vi "Config_LoadCreate.vi"(7 "Config In":path, 8 "error In":errorcluster, 10 "Configuration Cluster":T1={"General"={"Config.ini"=path "", "Default Logging Path"=path ""}, "Hardware"={"LCR VISA COM"="", "Measure Rate (1/s)"=0, "Reset on Load?"=FALSE, "Measure Profile"=path ""}, "HM8118 Current Profile"={"Bias Profile"={" Bias Source (OFF)"=0, " Bias Type (Voltage)"=0, "Bias Level (0)"=0.0}, "Measurement Profile"={"Operation Mode (0: Auto)"=0, "Circuit Type (2: Auto)"=2, "Manual Range (1:Range 1 and 25 Ohms)"=1, "Auto Range (T: Enable)"=TRUE}, "Signal Profile"={"Frequency (1kHz)"=1000.0, "Measuring Voltage (1V)"=1.0}, "Integration Profile"={"Averaging (0: Off)"=0, "Averaging Number (2)"=2, "Time (100ms)"=100, "Rate (0: Fast)"=0}, "Trigger Profile"={"Trigger Mode (0: Continuous)"=0}}, "HM8118 New Profile"={"Bias Profile"={" Bias Source (OFF)"=0, " Bias Type (Voltage)"=0, "Bias Level (0)"=0.0}, "Measurement Profile"={"Operation Mode (0: Auto)"=0, "Circuit Type (2: Auto)"=2, "Manual Range (1:Range 1 and 25 Ohms)"=1, "Auto Range (T: Enable)"=TRUE}, "Signal Profile"={"Frequency (1kHz)"=1000.0, "Measuring Voltage (1V)"=1.0}, "Integration Profile"={"Averaging (0: Off)"=0, "Averaging Number (2)"=2, "Time (100ms)"=100, "Rate (0: Fast)"=0}, "Trigger Profile"={"Trigger Mode (0: Continuous)"=0}}, "Operation"={"Operation Mode"=enum."Logging", "Status"=""}} {"HM8118 New Profile"."Trigger Profile"."Trigger Mode (0: Continuous)" items=["Continuous", "Manual", "External"]; "HM8118 New Profile"."Integration Profile"."Rate (0: Fast)" items=["Fast", "Medium", "Slow"]; "HM8118 New Profile"."Integration Profile"."Time (100ms)" min=1 max=999; "HM8118 New Profile"."Integration Profile"."Averaging Number (2)" min=2 max=99; "HM8118 New Profile"."Integration Profile"."Averaging (0: Off)" items=["Off", "Normal", "Averaging"]; "HM8118 New Profile"."Signal Profile"."Measuring Voltage (1V)" min=0.05 max=1.5 step=0.01; "HM8118 New Profile"."Signal Profile"."Frequency (1kHz)" min=20.0 max=200000.0; "HM8118 New Profile"."Measurement Profile"."Manual Range (1:Range 1 and 25 Ohms)" items=["Range 1 and 25 Ohms"=1, "Range 2 and 25 Ohms"=2, "Range 3 and 400 Ohms"=3, "Range 4 and 6.4 kOhms"=4, "Range 5 and 100kOhms"=5, "Range 6 and 100kOhms"=6]; "HM8118 New Profile"."Measurement Profile"."Circuit Type (2: Auto)" items=["Series", "Parallel", "Auto"]; "HM8118 New Profile"."Measurement Profile"."Operation Mode (0: Auto)" items=["Auto", "L+Q", "L+R", "C+D", "C+R", "R+Q", "Z+Theta", "Y+Theta", "R+X", "G+B", "N+Theta", "M"]; "HM8118 New Profile"."Bias Profile"."Bias Type (Voltage)" items=["Voltage", "Current"]; "HM8118 New Profile"."Bias Profile"."Bias Source (OFF)" items=["Off", "Internal", "External"]; "HM8118 Current Profile"."Trigger Profile"."Trigger Mode (0: Continuous)" items=["Continuous", "Manual", "External"]; "HM8118 Current Profile"."Integration Profile"."Rate (0: Fast)" items=["Fast", "Medium", "Slow"]; "HM8118 Current Profile"."Integration Profile"."Time (100ms)" min=1 max=999; "HM8118 Current Profile"."Integration Profile"."Averaging Number (2)" min=2 max=99; "HM8118 Current Profile"."Integration Profile"."Averaging (0: Off)" items=["Off", "Normal", "Averaging"]; "HM8118 Current Profile"."Signal Profile"."Measuring Voltage (1V)" min=0.05 max=1.5 step=0.01; "HM8118 Current Profile"."Signal Profile"."Frequency (1kHz)" min=20.0 max=200000.0; "HM8118 Current Profile"."Measurement Profile"."Manual Range (1:Range 1 and 25 Ohms)" items=["Range 1 and 25 Ohms"=1, "Range 2 and 25 Ohms"=2, "Range 3 and 400 Ohms"=3, "Range 4 and 6.4 kOhms"=4, "Range 5 and 100kOhms"=5, "Range 6 and 100kOhms"=6]; "HM8118 Current Profile"."Measurement Profile"."Circuit Type (2: Auto)" items=["Series", "Parallel", "Auto"]; "HM8118 Current Profile"."Measurement Profile"."Operation Mode (0: Auto)" items=["Auto", "L+Q", "L+R", "C+D", "C+R", "R+Q", "Z+Theta", "Y+Theta", "R+X", "G+B", "N+Theta", "M"]; "HM8118 Current Profile"."Bias Profile"."Bias Type (Voltage)" items=["Voltage", "Current"]; "HM8118 Current Profile"."Bias Profile"."Bias Source (OFF)" items=["Off", "Internal", "External"]}, 11 "LCR VISA COM":refnum<visa-resource-name>) -> (0 "error out":errorcluster, 2 "Configuration Cluster Out":T1={"General"={"Config.ini"=path "", "Default Logging Path"=path ""}, "Hardware"={"LCR VISA COM"="", "Measure Rate (1/s)"=0, "Reset on Load?"=FALSE, "Measure Profile"=path ""}, "HM8118 Current Profile"={"Bias Profile"={" Bias Source (OFF)"=0, " Bias Type (Voltage)"=0, "Bias Level (0)"=0.0}, "Measurement Profile"={"Operation Mode (0: Auto)"=0, "Circuit Type (2: Auto)"=2, "Manual Range (1:Range 1 and 25 Ohms)"=1, "Auto Range (T: Enable)"=TRUE}, "Signal Profile"={"Frequency (1kHz)"=1000.0, "Measuring Voltage (1V)"=1.0}, "Integration Profile"={"Averaging (0: Off)"=0, "Averaging Number (2)"=2, "Time (100ms)"=100, "Rate (0: Fast)"=0}, "Trigger Profile"={"Trigger Mode (0: Continuous)"=0}}, "HM8118 New Profile"={"Bias Profile"={" Bias Source (OFF)"=0, " Bias Type (Voltage)"=0, "Bias Level (0)"=0.0}, "Measurement Profile"={"Operation Mode (0: Auto)"=0, "Circuit Type (2: Auto)"=2, "Manual Range (1:Range 1 and 25 Ohms)"=1, "Auto Range (T: Enable)"=TRUE}, "Signal Profile"={"Frequency (1kHz)"=1000.0, "Measuring Voltage (1V)"=1.0}, "Integration Profile"={"Averaging (0: Off)"=0, "Averaging Number (2)"=2, "Time (100ms)"=100, "Rate (0: Fast)"=0}, "Trigger Profile"={"Trigger Mode (0: Continuous)"=0}}, "Operation"={"Operation Mode"=enum."Logging", "Status"=""}} {"HM8118 New Profile"."Trigger Profile"."Trigger Mode (0: Continuous)" items=["Continuous", "Manual", "External"]; "HM8118 New Profile"."Integration Profile"."Rate (0: Fast)" items=["Fast", "Medium", "Slow"]; "HM8118 New Profile"."Integration Profile"."Time (100ms)" min=1 max=999; "HM8118 New Profile"."Integration Profile"."Averaging Number (2)" min=2 max=99; "HM8118 New Profile"."Integration Profile"."Averaging (0: Off)" items=["Off", "Normal", "Averaging"]; "HM8118 New Profile"."Signal Profile"."Measuring Voltage (1V)" min=0.05 max=1.5 step=0.01; "HM8118 New Profile"."Signal Profile"."Frequency (1kHz)" min=20.0 max=200000.0; "HM8118 New Profile"."Measurement Profile"."Manual Range (1:Range 1 and 25 Ohms)" items=["Range 1 and 25 Ohms"=1, "Range 2 and 25 Ohms"=2, "Range 3 and 400 Ohms"=3, "Range 4 and 6.4 kOhms"=4, "Range 5 and 100kOhms"=5, "Range 6 and 100kOhms"=6]; "HM8118 New Profile"."Measurement Profile"."Circuit Type (2: Auto)" items=["Series", "Parallel", "Auto"]; "HM8118 New Profile"."Measurement Profile"."Operation Mode (0: Auto)" items=["Auto", "L+Q", "L+R", "C+D", "C+R", "R+Q", "Z+Theta", "Y+Theta", "R+X", "G+B", "N+Theta", "M"]; "HM8118 New Profile"."Bias Profile"."Bias Type (Voltage)" items=["Voltage", "Current"]; "HM8118 New Profile"."Bias Profile"."Bias Source (OFF)" items=["Off", "Internal", "External"]; "HM8118 Current Profile"."Trigger Profile"."Trigger Mode (0: Continuous)" items=["Continuous", "Manual", "External"]; "HM8118 Current Profile"."Integration Profile"."Rate (0: Fast)" items=["Fast", "Medium", "Slow"]; "HM8118 Current Profile"."Integration Profile"."Time (100ms)" min=1 max=999; "HM8118 Current Profile"."Integration Profile"."Averaging Number (2)" min=2 max=99; "HM8118 Current Profile"."Integration Profile"."Averaging (0: Off)" items=["Off", "Normal", "Averaging"]; "HM8118 Current Profile"."Signal Profile"."Measuring Voltage (1V)" min=0.05 max=1.5 step=0.01; "HM8118 Current Profile"."Signal Profile"."Frequency (1kHz)" min=20.0 max=200000.0; "HM8118 Current Profile"."Measurement Profile"."Manual Range (1:Range 1 and 25 Ohms)" items=["Range 1 and 25 Ohms"=1, "Range 2 and 25 Ohms"=2, "Range 3 and 400 Ohms"=3, "Range 4 and 6.4 kOhms"=4, "Range 5 and 100kOhms"=5, "Range 6 and 100kOhms"=6]; "HM8118 Current Profile"."Measurement Profile"."Circuit Type (2: Auto)" items=["Series", "Parallel", "Auto"]; "HM8118 Current Profile"."Measurement Profile"."Operation Mode (0: Auto)" items=["Auto", "L+Q", "L+R", "C+D", "C+R", "R+Q", "Z+Theta", "Y+Theta", "R+X", "G+B", "N+Theta", "M"]; "HM8118 Current Profile"."Bias Profile"."Bias Type (Voltage)" items=["Voltage", "Current"]; "HM8118 Current Profile"."Bias Profile"."Bias Source (OFF)" items=["Off", "Internal", "External"]}, 3 "LCR VISA COM Out":refnum<visa-resource-name>)   [LabVIEW 2021]
uses:
  Config_Cluster.ctl
  Mode_Enum.ctl
  <vilib>/Utility/config.llb/Read Key (Path).vi
  <vilib>/Utility/config.llb/NI_LVConfig.lvlib
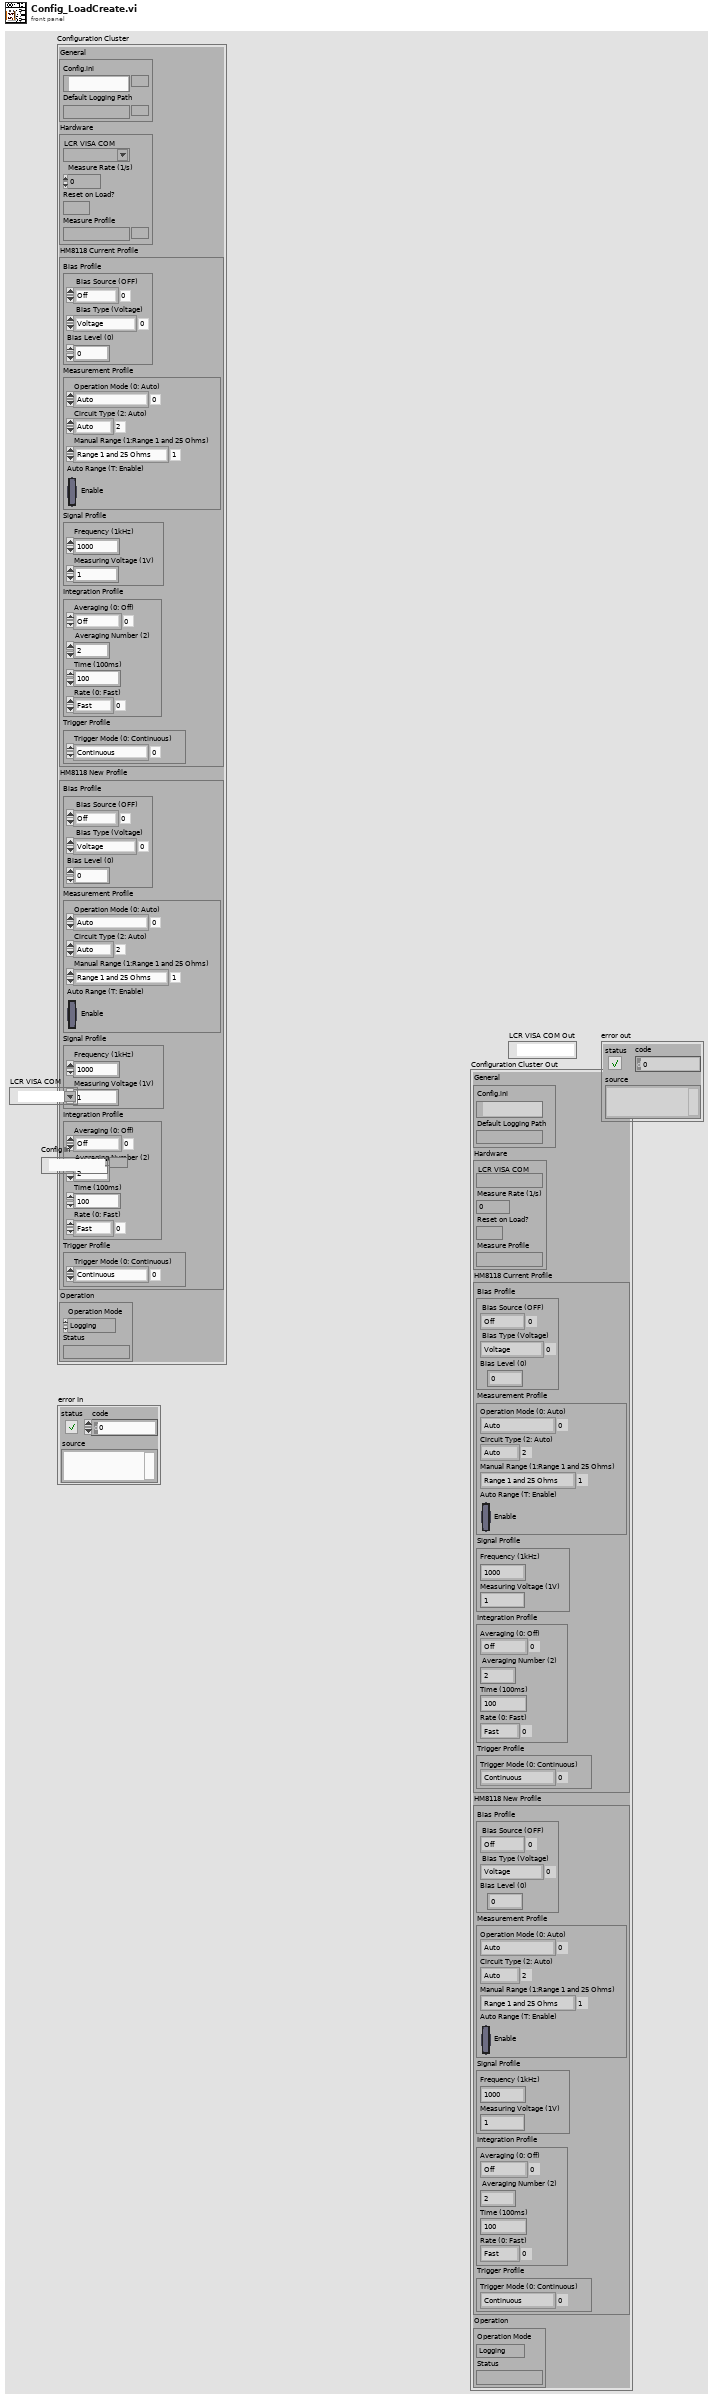
[diagram p1: front panel]
types:
  T1 = typedef "Config_Cluster.ctl" = cluster{"General":cluster{"Config.ini":path, "Default Logging Path":path}, "Hardware":cluster{"LCR VISA COM":refnum<visa-resource-name>, "Measure Rate (1/s)":i32, "Reset on Load?":bool, "Measure Profile":path}, "HM8118 Current Profile":cluster{"Bias Profile":cluster{" Bias Source (OFF)":u8, " Bias Type (Voltage)":u8, "Bias Level (0)":dbl}, "Measurement Profile":cluster{"Operation Mode (0: Auto)":u16, "Circuit Type (2: Auto)":u16, "Manual Range (1:Range 1 and 25 Ohms)":u8, "Auto Range (T: Enable)":bool}, "Signal Profile":cluster{"Frequency (1kHz)":dbl, "Measuring Voltage (1V)":dbl}, "Integration Profile":cluster{"Averaging (0: Off)":u16, "Averaging Number (2)":i32, "Time (100ms)":i32, "Rate (0: Fast)":u16}, "Trigger Profile":cluster{"Trigger Mode (0: Continuous)":u16}}, "HM8118 New Profile":cluster{"Bias Profile":cluster{" Bias Source (OFF)":u8, " Bias Type (Voltage)":u8, "Bias Level (0)":dbl}, "Measurement Profile":cluster{"Operation Mode (0: Auto)":u16, "Circuit Type (2: Auto)":u16, "Manual Range (1:Range 1 and 25 Ohms)":u8, "Auto Range (T: Enable)":bool}, "Signal Profile":cluster{"Frequency (1kHz)":dbl, "Measuring Voltage (1V)":dbl}, "Integration Profile":cluster{"Averaging (0: Off)":u16, "Averaging Number (2)":i32, "Time (100ms)":i32, "Rate (0: Fast)":u16}, "Trigger Profile":cluster{"Trigger Mode (0: Continuous)":u16}}, "Operation":cluster{"Operation Mode":T2, "Status":string}}
  T2 = typedef "Mode_Enum.ctl" = enum16{"Logging", "Idle-Off", "Idle"}
  T3 = typedef "NI_LVConfig.lvlib/Config Data RefNum.ctl" = refnum<k1>
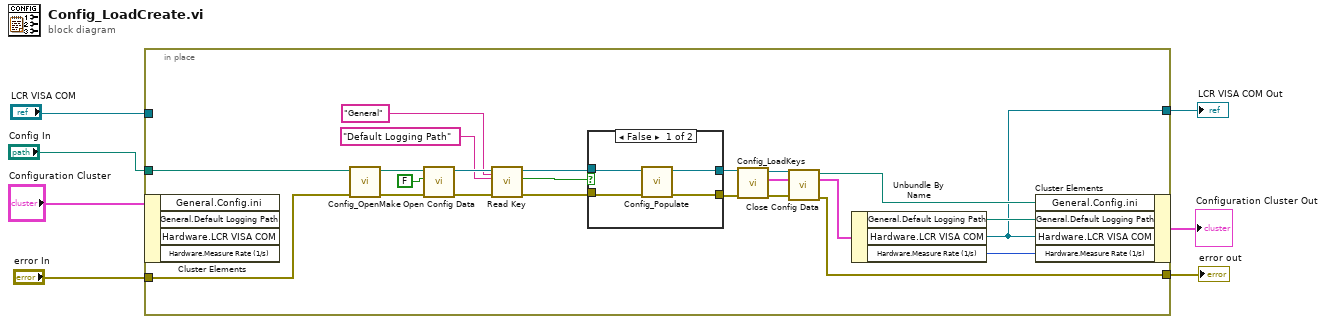
[diagram p0: block diagram]
diagram:
  n1 = in-place {
    in-place-border: "LCR VISA COM" -> [_]
    in-place-border: "error In" -> [w28]
    in-place-border: "Config In" -> [w29]
    in-place-border: [w9] -> w3
    in-place-border: [w8] -> w1
    n2 = in-place-cluster #1("Configuration Cluster") -> ()  [unwired: 4 out]
    n3 = call "Config_OpenMake.vi"("error in (no error)"=w28, "Config Path"=w29) -> ("error out"=w25:errorcluster, "File Path"=w27:path)  [unwired: 8 in]
    n4 = call <vilib>:"Open Config Data.vi"("error in (no error)"=w25, "create file if necessary (T)"=FALSE, "configuration file path"=w27) -> ("error out"=w23:errorcluster, "refnum"=w24:T3)  [unwired: 6 in, 1 out]
    n5 = call-poly <vilib>:"Read Key.vi"("section"="General", "error in (no error)"=w23, "key"="Default Logging Path", "refnum"=w24) -> ("error out"=w19:errorcluster, "found?"=w18:bool, "refnum out"=w20:T3)  [unwired: 4 in, 1 out]
    n6 = case shown="False" w18 {
      tunnel: w19 -> [w32 w34]
      tunnel: w20 -> [w33 w35]
      tunnel: [w31 w34] -> w14
      tunnel: [w30 w35] -> w16
      frame False {
        n7 = call "Config_Populate.vi"("error in (no error)"=w32, "Config Ref In"=w33) -> ("error out"=w31:errorcluster, "refnum out"=w30:T3)  [unwired: 8 in]
      }
      frame True {
      }
    }
    n8 = call "Config_LoadKeys.vi"("error in (no error)"=w14, "Config In"=w16) -> ("error out"=w13:errorcluster, "output cluster"=w12:T1, "refnum out"=w15:T3)  [unwired: 7 in]
    n9 = call <vilib>:"Close Config Data.vi"("error in (no error)"=w13, "refnum"=w15) -> ("error out"=w8:errorcluster, "file path"=w17:path)  [unwired: 8 in]
    n10 = Unbundle By Name(w12) -> ("General.Default Logging Path"=w11:path, "Hardware.LCR VISA COM"=w9:refnum<visa-resource-name>, "Hardware.Measure Rate (1/s)"=w10:i32)
    n11 = in-place-cluster #1("General.Config.ini"=w17, "General.Default Logging Path"=w11, "Hardware.LCR VISA COM"=w9, "Hardware.Measure Rate (1/s)"=w10) -> (→"Configuration Cluster Out":T1)
  }
  "LCR VISA COM Out" <- w3
  "error out" <- w1
